vi "Set ID.vi"(8 "pID":T1, 11 "iCameraID":i32) -> (0 "pID out":T1, 3 "function return":i32)   [LabVIEW 2012, in "LV_swapper.lvlib"]
doc: "__declspec(dllexport) ASI_ERROR_CODE SetID(int iCameraID, ASI_ID* pID);"
uses:
  <userlib>/LV_swapper/LV_swapper.lvlib
  <userlib>/LV_swapper/LV_swapper.dll
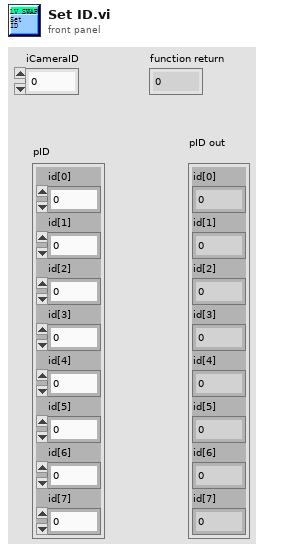
[diagram p1: front panel]
types:
  T1 = cluster{"id[0]":u8, "id[1]":u8, "id[2]":u8, "id[3]":u8, "id[4]":u8, "id[5]":u8, "id[6]":u8, "id[7]":u8}
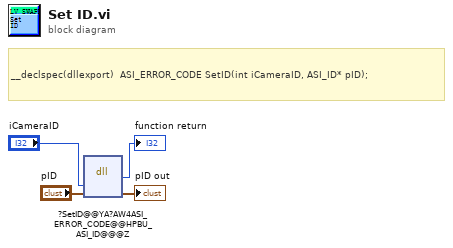
[diagram p0: block diagram]
diagram:
  # "__declspec(dllexport)  ASI_ERROR_CODE SetID(int iCameraID, ASI_ID* pID);"
  n1 = dll-call lib="D:/Program Files (x86)/National Instruments/LabVIEW 2012/user.lib/LV_swapper/LV_swapper.*" fn="?SetID@@YA?AW4ASI_ERROR_CODE@@HPBU_ASI_ID@@@Z"("iCameraID"="iCameraID", "pID"="pID") -> ("返回类型"=→"function return":i32, "pID"=→"pID out":T1)  [unwired: 4 in, 2 out]
